vi "Sub_Accel_Volt2ms2.vi"(11 "ACC volts":dbl[](array[numeric])) -> (3 "ACC m/s2":dbl[](array[numeric]))   [LabVIEW 2019]
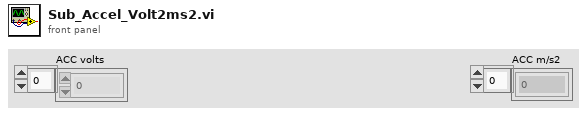
[diagram p1: front panel]
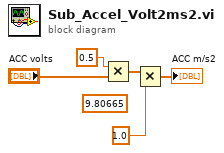
[diagram p0: block diagram]
diagram:
  (unwired) 9.80665
  n1 = Multiply(x=0.5, y="ACC volts") -> (x*y=w5:dbl[])
  n2 = Multiply(x=w5, y=1.0) -> (x*y=→"ACC m/s2":dbl[])
